vi "Global Settings.vi"(8 "error in (no error)":errorcluster, 11 "Node Ptr":T1 format="%.0x") -> (0 "error out":errorcluster)   [LabVIEW 2019, in "Fuel Injector Analysis Addon System Explorer.lvlib"]
uses:
  Fuel Injector Analysis Addon System Explorer.lvlib
  <vilib>/NI VeriStand/Custom Device API/Custom Device Item Ref.ctl
  Addon Shared/SubVIs/Constants.vi
  <vilib>/NI VeriStand/Custom Device API/Get Item Property (Double).vi
  <vilib>/NI VeriStand/Custom Device API/Set Item Property (Double).vi
  <vilib>/NI VeriStand/Custom Device API/Custom Device API.lvlib
  Addon Shared/Fuel Injector Analysis Addon Shared.lvlib
panel:
  in  "Multicolumn Listbox":i32(listbox)
  in  "SHDocVw.IWebBrowser":refnum<k7>(container)
  in  "Description":string
  in  "Timeout (seconds)":dbl=5.0
  in  "Header":cluster{"Section Name":string}={"Section Name"="Custom Device Item Settings"}
  in  "Name":string
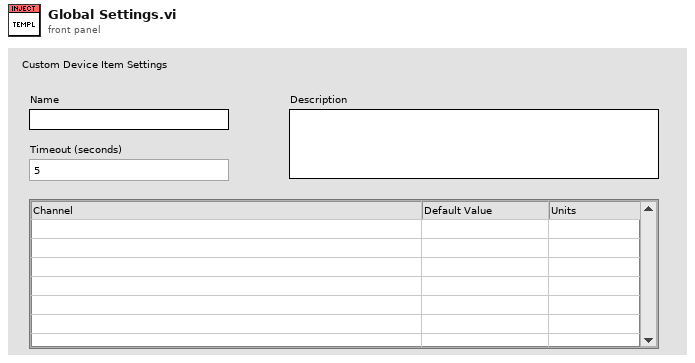
[diagram p1: front panel]
types:
  T1 = typedef "Custom Device API.lvlib/Custom Device Item Ref.ctl" = u64
  T2 = typedef "Custom Device API.lvlib/Custom Device Item Info.ctl" = cluster{"Name":string, "Is Channel":bool, "GUID":string, "Is Waveform":bool}
  T3 = typedef "Custom Device API.lvlib/Custom Device Channel.ctl" = cluster{"Type":T4, "Units":string, "Default Value":dbl, "Faultable":bool, "Scalable":bool}
  T4 = typedef "Custom Device API.lvlib/Custom Device Channel Type.ctl" = enum16{"Input", "Output"}
  T5 = typedef "Custom Device API.lvlib/Custom Device Commands.ctl" = enum16{"Default", "Item renamed", "Shutdown", "Dynamic button pressed"}
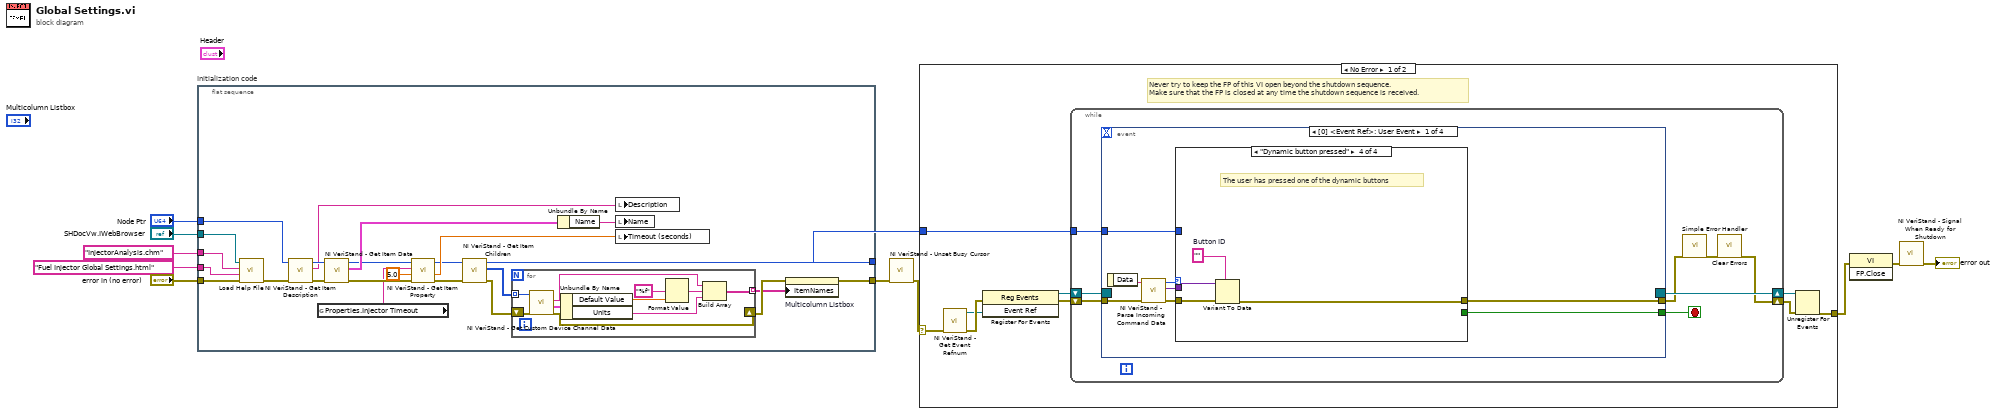
[diagram p0: block diagram]
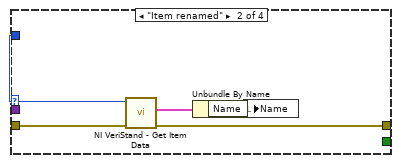
[diagram p3: hidden frame]
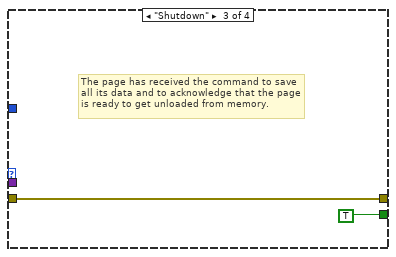
[diagram p4: hidden frame]
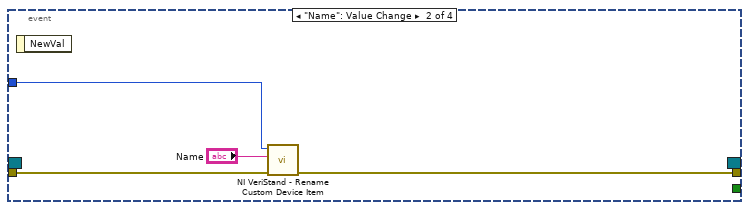
[diagram p5: hidden frame]
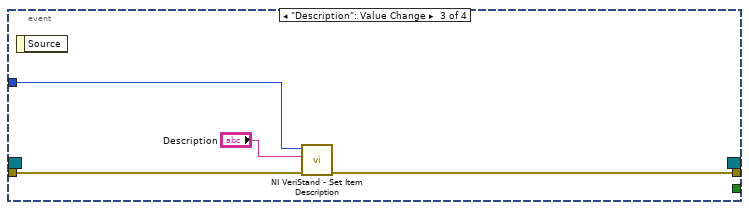
[diagram p6: hidden frame]
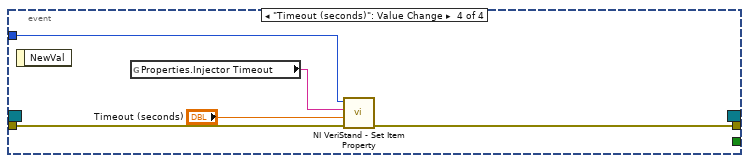
[diagram p7: hidden frame]
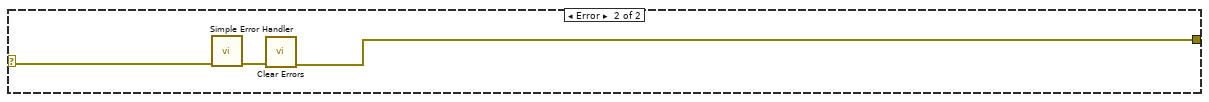
[diagram p8: hidden frame]
diagram:
  n1 = flat-sequence "Initialization code" {
    tunnel: "error in (no error)" -> [w28]
    tunnel: "Node Ptr" -> [w34]
    tunnel: [w12] -> w7
    tunnel: [w18] -> w4
    tunnel: "Fuel Injector Global Settings.html" ("HTML File") -> [w27]
    tunnel: "InjectorAnalysis.chm" ("Main CHM File") -> [w26]
    tunnel: "SHDocVw.IWebBrowser" -> [w25]
    frame #0 {
      n2 = call "Load Help File.vi"("error in (no error)"=w28, "HTML File"=w27, "Main CHM File"=w26, "SHDocVw.IWebBrowser2"=w25) -> ("error out"=w29:errorcluster)  [unwired: 7 in]
      n3 = call <vilib>:"NI VeriStand - Get Item Description.vi"("error in (no error)"=w29, "Item Ref in"=w34) -> ("error out"=w33:errorcluster, "Description"=w30:string, "Item Ref out"=w35:T1)  [unwired: 7 out]
      n4 = global read "Constants.vi" "Properties.Injector Timeout"() -> (w19:string)
      n5 = call <vilib>:"NI VeriStand - Get Item Data.vi"("error in (no error)"=w33, "Item Ref in"=w35) -> ("error out"=w24:errorcluster, "Item Info"=w32:T2, "Item Ref out"=w23:T1)  [unwired: 7 out]
      n6 = call-poly <vilib>:"NI VeriStand - Get Item Property.vi"("error in (no error)"=w24, "Default Value"=5.0, "Property Name"=w19, "Item Ref in"=w23) -> ("error out"=w17:errorcluster, "Value"=w21:dbl, "Item Ref out"=w20:T1)  [unwired: 4 in, 1 out]
      n7 = call <vilib>:"NI VeriStand - Get Item Children.vi"("error in (no error)"=w17, "Item Ref in"=w20) -> ("error out"=w16:errorcluster, "Child Refs"=w15:T1[], "Item Ref out"=w18:T1)  [unwired: 6 in, 1 out]
      n8 = for {
        tunnel: w15 -> [w45] mode=indexing
        tunnel: [w37] -> w13 mode=indexing
        shift-right: [w36] -> w14
        shift-left: w16 -> [w44]
        n9 = call <vilib>:"NI VeriStand - Get Custom Device Channel Data.vi"("error in (no error)"=w44, "Channel Ref in"=w45) -> ("error out"=w36:errorcluster, "Channel"=w43:T3, "Channel Name"=w38:string)  [unwired: 4 in, 3 out]
        n10 = Unbundle By Name(w43) -> ("Default Value"=w42:dbl, "Units"=w40:string)
        n11 = Format Value(format string="%f", value (0)=w42) -> (output string=w39:string)  [unwired: 1 in]
        n12 = Build Array(w38, w39, w40) -> (w37:string[])
      }
      n13 = Unbundle By Name(w32) -> ("Name"=w31:string)
      n14 = local write "Description"(w30) -> ()
      n15 = local write "Name"(w31) -> ()
      n16 = local write "Timeout (seconds)"(w21) -> ()
      n17 = property on="Multicolumn Listbox" class="MCListbox (strict)"(error in=w14, "ItemNames"=w13) -> (error out=w12:errorcluster)  [unwired: 1 in, 1 out]
    }
  }
  n18 = call <vilib>:"NI VeriStand - Unset Busy Cursor.vi"("error in (no error)"=w7) -> ("error out"=w6:errorcluster)  [unwired: 10 out]
  n19 = case shown="No Error" w6 {
    selector: w6 -> [w46 w98]
    tunnel: [w51 w96] -> w11
    tunnel: w4 -> [w47 _]
    frame No Error {
      # "Never try to keep the FP of this VI open beyond the shutdown sequence.\nMake sure that the FP is closed at any time the shutdown sequence is received."
      n20 = call <vilib>:"NI VeriStand - Get Event Refnum.vi"("error in (no error)"=w46) -> ("error out"=w54:errorcluster, "Event Ref"=w50:refnum<user-event>)  [unwired: 9 out]
      n21 = register-events(error in=w54, w50) -> (reference out=w48:refnum<event-registration>, error out=w49:errorcluster)  [unwired: 1 in]
      n22 = while {
        tunnel: w47 -> [w58]
        shift-right: [w55] -> w52
        shift-left: w49 -> [w61]
        shift-right: [w62] -> w53
        shift-left: w48 -> [w60]
        stop <- w59 stop-if-true
        n23 = event shown="[0] <Event Ref>: User Event" {
          selector: w60 -> [_ _ _ _]
          dyn-events: [_ _ _ _] -> w62
          timeout: _ -> [_ _ _ _]
          tunnel: w61 -> [w70 w86 w90 w95]
          tunnel: [w66 _ _ _] -> w59
          tunnel: [w65 w85 w87 w94] -> w57
          tunnel: w58 -> [w64 w84 w89 w93]
          event User Event {
            n24 = event-data() -> ("Data"=w69:string)  [unwired: 1 out]
            n25 = call <vilib>:"NI VeriStand - Parse Incoming Command Data.vi"("error in (no error)"=w70, "Incoming data"=w69) -> ("error out"=w68:errorcluster, "Outgoing data"=w63:variant, "Action"=w67:T5)  [unwired: 7 out]
            n26 = case shown="\"Dynamic button pressed\"" w67 {
              tunnel: w68 -> [w71 w76 w77 w82]
              tunnel: [_ _ TRUE _] -> w66
              tunnel: [w71 w73 w77 w79] -> w65
              tunnel: w64 -> [_ w75 _ _]
              tunnel: w63 -> [_ _ _ w81]
              frame "Default", Default {
              }
              frame "Item renamed" {
                n27 = call <vilib>:"NI VeriStand - Get Item Data.vi"("error in (no error)"=w76, "Item Ref in"=w75) -> ("error out"=w73:errorcluster, "Item Info"=w74:T2)  [unwired: 8 out]
                n28 = Unbundle By Name(w74) -> ("Name"=w72:string)
                n29 = local write "Name"(w72) -> ()
              }
              frame "Shutdown" {
                # "The page has received the command to save all its data and to acknowledge that the page is ready to get unloaded from memory."
              }
              frame "Dynamic button pressed" {
                w80 = ""  # Button ID
                # "The user has pressed one of the dynamic buttons"
                n30 = Variant To Data(error in=w82, type=w80, Variant=w81) -> (error out=w79:errorcluster)  [unwired: 1 out]
              }
            }
          }
          event "Name": Value Change {
            n31 = event-data() -> ()  [unwired: 2 out]
            n32 = call <vilib>:"NI VeriStand - Rename Custom Device Item.vi"("error in (no error)"=w86, "New Name"="Name", "Item Ref in"=w84) -> ("error out"=w85:errorcluster)  [unwired: 1 in, 7 out]
          }
          event "Description": Value Change {
            n33 = event-data() -> ()  [unwired: 2 out]
            n34 = call <vilib>:"NI VeriStand - Set Item Description.vi"("error in (no error)"=w90, "Description"="Description", "Item Ref in"=w89) -> ("error out"=w87:errorcluster)  [unwired: 6 in, 2 out]
          }
          event "Timeout (seconds)": Value Change {
            n35 = event-data() -> ()  [unwired: 2 out]
            n36 = global read "Constants.vi" "Properties.Injector Timeout"() -> (w91:string)
            n37 = call-poly <vilib>:"NI VeriStand - Set Item Property.vi"("error in (no error)"=w95, "Value"="Timeout (seconds)", "Property Name"=w91, "Item Ref in"=w93) -> ("error out"=w94:errorcluster)  [unwired: 5 in, 2 out]
          }
        }
        n38 = call <vilib>:"Simple Error Handler.vi"("error in (no error)"=w57) -> ("error out"=w56:errorcluster)  [unwired: 1 in, 7 out]
        n39 = call <vilib>:"Clear Errors.vi"("error in (no error)"=w56) -> ("error out"=w55:errorcluster)  [unwired: 1 in, 5 out]
      }
      n40 = Unregister For Events(event registration refnum=w53, error in=w52) -> (error out=w51:errorcluster)
    }
    frame Error {
      n41 = call <vilib>:"Simple Error Handler.vi"("error in (no error)"=w98) -> ("error out"=w97:errorcluster)  [unwired: 1 in, 7 out]
      n42 = call <vilib>:"Clear Errors.vi"("error in (no error)"=w97) -> ("error out"=w96:errorcluster)  [unwired: 1 in, 5 out]
    }
  }
  n43 = invoke class="VI" method="FP.Close"(error in=w11) -> (error out=w10:errorcluster)  [unwired: 2 in, 2 out]
  n44 = call <vilib>:"NI VeriStand - Signal When Ready for Shutdown.vi"("error in (no error)"=w10) -> ("error out"=→"error out":errorcluster)  [unwired: 10 out]
